vi "Emballage_BDD_CC_Dagmar_S1220009.vi"(7 "Temps imprimante":dbl=3.0 caption="Attente (s)", 8 "entrée d'erreur":errorcluster caption="entrée d'erreur (pas d'erreur)", 9 "SN_Bloc 2":string, 10 "donnée":string[](array[string]), 11 "chemin":path=path "\\\\Plz-inf-nas\\mtd_prd_tests/PARAM_TESTS/PROD_Data-Admin/M1200217b.doc") -> (0 "sortie d'erreur":errorcluster)   [LabVIEW 2020]
uses:
  Modules/FS/60_FS_Controles/60_FS_SetGet.ctl
panel:
  out "Date_test":string
  out "SN_Bloc":string
  out "SN_Revol.TG":string
  out "SN_Revol.O2":string
  out "Indice_Bloc":string
  out "Indice_Revol.TG":string
  out "Indice_Revol.O2":string
  out "Tab_Text":string[](array[string])=["22 / 03 / 2010", "06", "ASBB5058", "08", "08", "ASBB2051", "ASBB2052"]
  in  "Tab_Names":string[](array[string])=["Date_Test", "Index_Bloc", "N_Série_Bloc", "Index_Revolver_O2", "Index_Revolver_TG", "N_Série_Revolver_O2", "N_Série_Revolver_TG"]
  in  "Word._Application":refnum<k7>
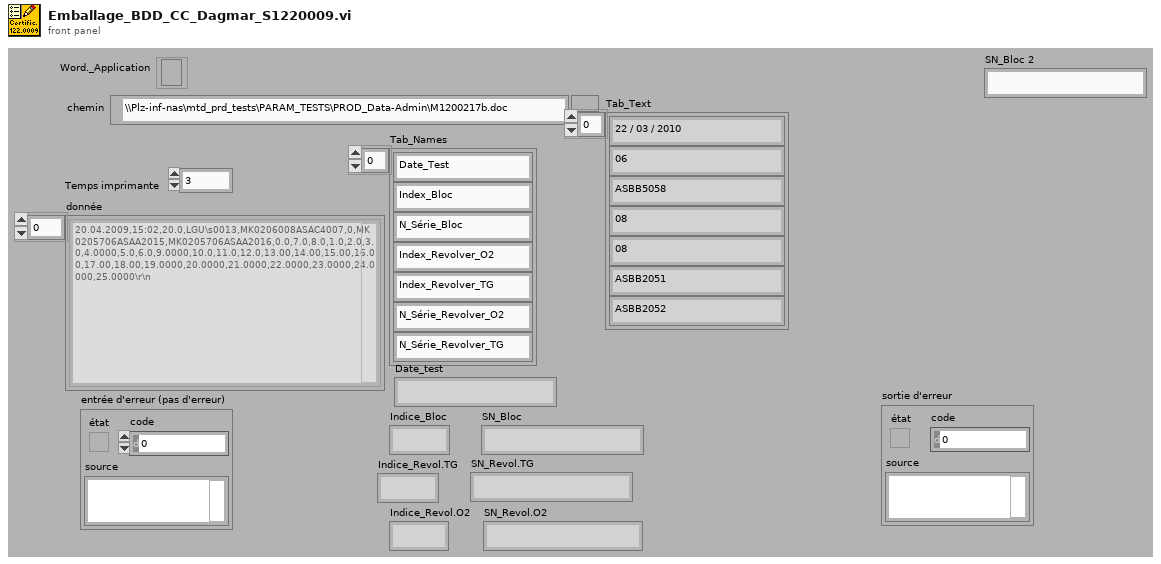
[diagram p1: front panel]
types:
  T1 = typedef "60_FS_SetGet.ctl" = enum16{"set", "get"}
  T2 = typedef "60_FS_CLT_Chemins.ctl" = cluster{"Racine_local":path, "Racine_reseau":path, "Racine_Support_Application":path, "Fichier_Journalisation":path, "Connexion_BDD_VSX":path, "Connexion_BDD_PLZ":path}
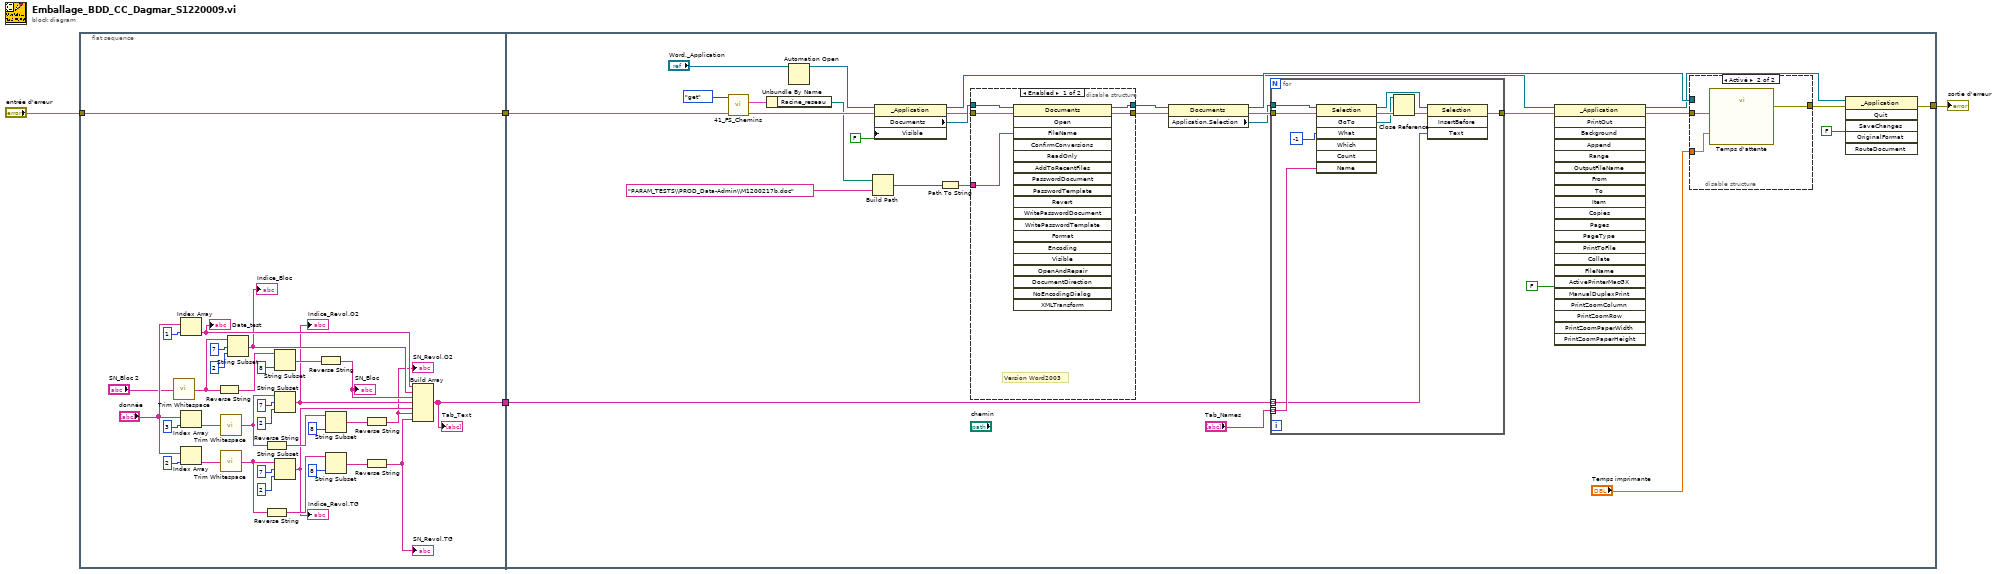
[diagram p0: block diagram]
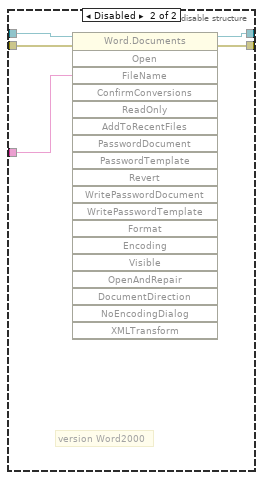
[diagram p2: hidden frame]
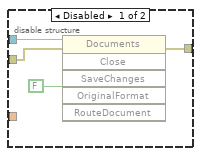
[diagram p3: hidden frame]
diagram:
  n1 = flat-sequence {
    tunnel: "entrée d'erreur" -> [w18]
    tunnel: [w18] -> w2
    tunnel: [w10] -> w1
    tunnel: [w52] -> w4
    tunnel: w2 -> [w45]
    tunnel: w1 -> [w51]
    frame #0 {
      n2 = call <vilib>:"Trim Whitespace.vi"("string"="SN_Bloc 2") -> ("trimmed string"=w7:string)  [unwired: 1 in]
      n3 = Index Array(array="donnée", index=1 ("indice")) -> (element=w17:string)
      "Date_test" <- w17
      n4 = Index Array(array="donnée", index=3 ("indice")) -> (element=w28:string)
      n5 = Index Array(array="donnée", index=2 ("indice")) -> (element=w29:string)
      n6 = Reverse String(1:w7) -> (0:w27:string)
      n7 = call <vilib>:"Trim Whitespace.vi"("string"=w28) -> ("trimmed string"=w5:string)  [unwired: 1 in]
      n8 = call <vilib>:"Trim Whitespace.vi"("string"=w29) -> ("trimmed string"=w6:string)  [unwired: 1 in]
      n9 = String Subset(string=w7, offset (0)=7, length (rest)=2 ("longueur (reste)")) -> (substring=w16:string)
      "Indice_Bloc" <- w16
      n10 = Reverse String(1:w5) -> (0:w21:string)
      n11 = Reverse String(1:w6) -> (0:w23:string)
      n12 = String Subset(string=w27, length (rest)=8 ("longueur (reste)")) -> (substring=w25:string)  [unwired: 1 in]
      n13 = String Subset(string=w5, offset (0)=7, length (rest)=2 ("longueur (reste)")) -> (substring=w14:string)
      "Indice_Revol.O2" <- w14
      n14 = String Subset(string=w6, offset (0)=7, length (rest)=2 ("longueur (reste)")) -> (substring=w13:string)
      "Indice_Revol.TG" <- w13
      n15 = Reverse String(1:w25) -> (0:w15:string)
      "SN_Bloc" <- w15
      n16 = String Subset(string=w21, length (rest)=8 ("longueur (reste)")) -> (substring=w19:string)  [unwired: 1 in]
      n17 = String Subset(string=w23, length (rest)=8 ("longueur (reste)")) -> (substring=w20:string)  [unwired: 1 in]
      n18 = Reverse String(1:w19) -> (0:w12:string)
      "SN_Revol.O2" <- w12
      n19 = Reverse String(1:w20) -> (0:w11:string)
      "SN_Revol.TG" <- w11
      n20 = Build Array(w17, w16, w15, w14, w13, w12, w11) -> (w10:string[])
      "Tab_Text" <- w10
    }
    frame #1 {
      n21 = call "41_FS_Chemins.vi"("error in (no error)"=w45, "SetGet"=60_FS_SetGet."get") -> ("error out"=w44:errorcluster, "CLT_Chemins_out"=w42:T2)  [unwired: 8 in]
      n22 = Unbundle By Name(w42) -> ("Racine_reseau"=w41:path)
      n23 = Automation Open ("Automation Ouvrir")(Automation Refnum="Word._Application") -> (Automation Refnum=w66:refnum<k7>)  [unwired: 3 in, 1 out]
      n24 = Build Path(base path=w41, name or relative path="PARAM_TESTS\\PROD_Data-Admin\\M1200217b.doc" ("nom ou chemin relatif")) -> (appended path=w39:path)
      n25 = property class="_Application"(reference=w66, error in=w44, "Visible"=FALSE) -> (reference out=w55:refnum<k7>, error out=w46:errorcluster, "Documents"=w47:refnum<k7>)
      n26 = Path To String(path=w39) -> (string=w50:string)
      n27 = disable-structure shown="Enabled" {
        disable-tunnel: w50 -> [w72 w73]
        disable-tunnel: [w71 w77] -> w49
        disable-tunnel: [w70 w75] -> w48
        disable-tunnel: w47 -> [w69 w76]
        disable-tunnel: w46 -> [w68 w74]
        frame Enabled {
          # "Version Word2003"
          n28 = invoke class="Documents" method="Open"(reference=w69, error in=w68, "FileName"=w72) -> (reference out=w71:refnum<k7>, error out=w70:errorcluster)  [unwired: 16 in, 17 out]
        }
        frame Disabled {
          # "version Word2000"
          n29 = invoke class="Word.Documents" method="Open"(reference=w76, error in=w74, "FileName"=w73) -> (reference out=w77:refnum<k7>, error out=w75:errorcluster)  [unwired: 16 in, 17 out]
        }
      }
      n30 = property class="Documents"(reference=w49, error in=w48) -> (reference out=w58:refnum<k7>, error out=w61:errorcluster, "Application.Selection"=w60:refnum<k7>)
      n31 = for {
        tunnel: "Tab_Names" -> [w91] mode=indexing
        tunnel: w51 -> [w90] mode=indexing
        tunnel: w61 -> [w89]
        tunnel: w60 -> [w88]
        tunnel: [w87] -> w59
        n32 = invoke class="Selection" method="GoTo"(reference=w88, error in=w89, "What"=-1, "Name"=w91) -> (reference out=w86:refnum<k7>, error out=w94:errorcluster, "GoTo"=w85:refnum<k7>)  [unwired: 3 in, 4 out]
        n33 = Close Reference(reference=w85, error in (no error)=w94) -> (error out=w93:errorcluster)
        n34 = invoke class="Selection" method="InsertBefore"(reference=w86, error in=w93, "Text"=w90) -> (error out=w87:errorcluster)  [unwired: 1 in, 3 out]
      }
      n35 = invoke class="_Application" method="PrintOut"(reference=w55, error in=w59, "PrintToFile"=FALSE) -> (reference out=w54:refnum<k7>, error out=w64:errorcluster)  [unwired: 19 in, 20 out]
      n36 = disable-structure shown="Activé" {
        disable-tunnel: w64 -> [w80 w84]
        disable-tunnel: w58 -> [w79 _]
        disable-tunnel: [w78 w83] -> w57
        disable-tunnel: "Temps imprimante" -> [_ w82]
        frame Disabled {
          n37 = invoke class="Documents" method="Close"(reference=w79, error in=w80, "SaveChanges"=FALSE) -> (error out=w78:errorcluster)  [unwired: 3 in, 5 out]
        }
        frame Enabled {
          n38 = call "Temps d'attente"("error in (no error)"=w84, "Delay Time (s)"=w82) -> ("error out"=w83:errorcluster)  [unwired: 9 in]
        }
      }
      n39 = invoke class="_Application" method="Quit"(reference=w54, error in=w57, "SaveChanges"=FALSE) -> (error out=w52:errorcluster)  [unwired: 3 in, 5 out]
    }
  }
  "sortie d'erreur" <- w4
